vi "whichTable.vi"(1 "element":T1) -> (0 "String":string)   [LabVIEW 2011]
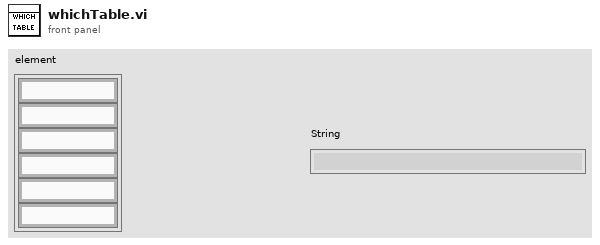
[diagram p1: front panel]
types:
  T1 = cluster{string, string, string, string, string, string}
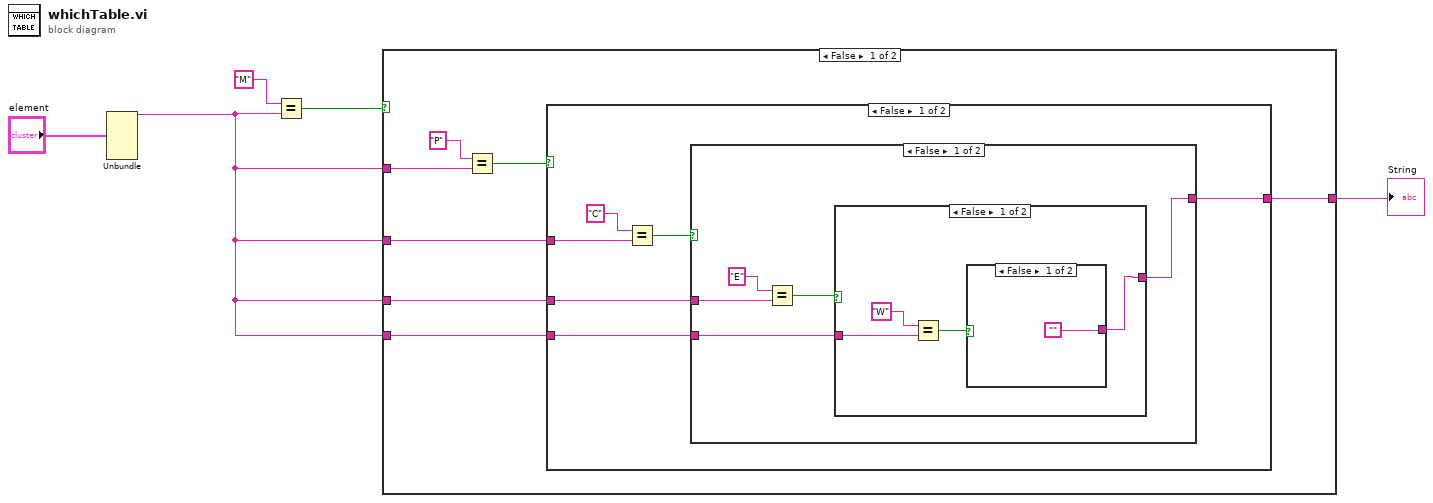
[diagram p0: block diagram]
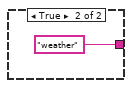
[diagram p2: hidden frame]
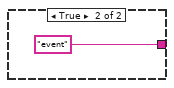
[diagram p3: hidden frame]
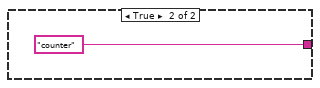
[diagram p4: hidden frame]
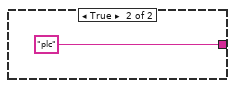
[diagram p5: hidden frame]
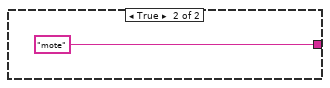
[diagram p6: hidden frame]
diagram:
  n1 = Unbundle("element") -> (w1:string)  [unwired: 5 out]
  n2 = Equal?(x="M", y=w1) -> (x = y?=w4:bool)
  n3 = case shown="False" w4 {
    tunnel: w1 -> [w10 _]
    tunnel: [w9 "mote" ("x")] -> w2
    tunnel: w1 -> [w8 _]
    tunnel: w1 -> [w7 _]
    tunnel: w1 -> [w6 _]
    frame False {
      n4 = Equal?(x="P", y=w10) -> (x = y?=w12:bool)
      n5 = case shown="False" w12 {
        tunnel: [w16 "plc" ("x")] -> w9
        tunnel: w8 -> [w17 _]
        tunnel: w7 -> [w14 _]
        tunnel: w6 -> [w13 _]
        frame False {
          n6 = Equal?(x="C", y=w17) -> (x = y?=w15:bool)
          n7 = case shown="False" w15 {
            tunnel: [w20 "counter" ("x")] -> w16
            tunnel: w14 -> [w22 _]
            tunnel: w13 -> [w19 _]
            frame False {
              n8 = Equal?(x="E", y=w22) -> (x = y?=w21:bool)
              n9 = case shown="False" w21 {
                tunnel: [w24 "event"] -> w20
                tunnel: w19 -> [w26 _]
                frame False {
                  n10 = Equal?(x="W", y=w26) -> (x = y?=w25:bool)
                  n11 = case shown="False" w25 {
                    tunnel: ["" "weather"] -> w24
                    frame False {
                    }
                    frame True {
                    }
                  }
                }
                frame True {
                }
              }
            }
            frame True {
            }
          }
        }
        frame True {
        }
      }
    }
    frame True {
    }
  }
  "String" <- w2
